vi "execute.vi"(8 "error in (no error)":errorcluster, 10 "Context in":refnum<class "Context.lvclass">, 11 "ManipulateM1M3Command in":refnum<class "ManipulateM1M3Command.lvclass">) -> (0 "error out":errorcluster, 2 "Context out":refnum<class "Context.lvclass">, 3 "ManipulateM1M3Command out":refnum<class "ManipulateM1M3Command.lvclass">)   [LabVIEW 2016, in "ManipulateM1M3Command.lvclass"]
uses:
  ManipulateM1M3Command.lvclass
  Context/Context.lvclass
  ManipulateM1M3Command.lvclass/ManipulateM1M3Command.ctl
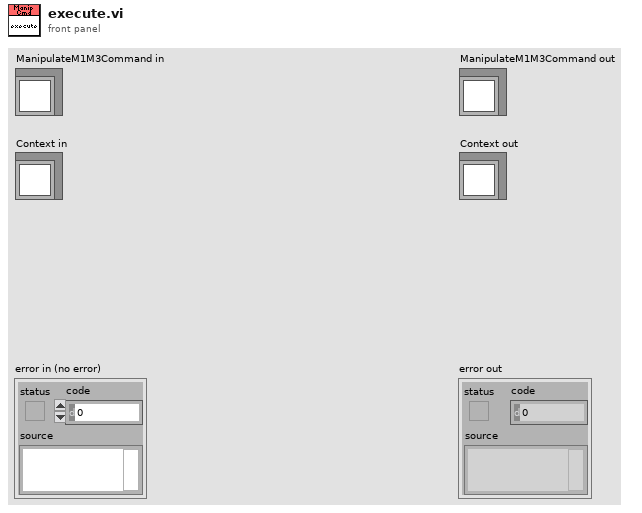
[diagram p1: front panel]
types:
  T1 = typedef "M1M3SupportTopics.lvlib/CommandManipulateM1M3.ctl" = cluster{"CommandId":T2, "XTranslation":dbl, "YTranslation":dbl, "ZTranslation":dbl, "XRotation":dbl, "YRotation":dbl, "ZRotation":dbl}
  T2 = typedef "M1M3SupportTopics.lvlib/CommandId.ctl" = i32
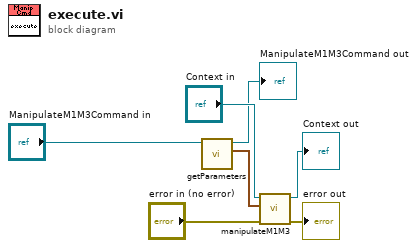
[diagram p0: block diagram]
diagram:
  n1 = call "getParameters.vi"("ManipulateM1M3Command in"="ManipulateM1M3Command in") -> ("Parameters"=w6:T1, "ManipulateM1M3Command out"=→"ManipulateM1M3Command out":refnum<class "ManipulateM1M3Command.lvclass">)  [unwired: 9 in]
  n2 = call-dynamic "manipulateM1M3.vi"("error in (no error)"="error in (no error)", "Parameters"=w6, "Context in"="Context in") -> ("error out"=→"error out":errorcluster, "Context out"=→"Context out":refnum<class "Context.lvclass">)  [unwired: 7 in]
